vi "Configure Channel Output.vi"(0 "VISA resource name":refnum<visa-resource-name>, 1 "Output Impedance (50 Ohm)":dbl=50.0, 2 "High Voltage Limit (5 V)":dbl=5.0, 3 "Output Polarity (0: Normal)":i32(ring) items=["Normal", "Inverted"], 5 "Channel (1: 1)":i32(ring)=1 items=["1"=1, "2"=2], 9 "Output State (0: Normal)":i32(ring) items=["Normal", "Gated"], 11 "error in (no error)":errorcluster, 12 "Enable Output (T: Enable)":bool=TRUE, 13 "Low Voltage Limit (-5 V)":dbl=-5.0, 14 "Enable Voltage Limit (T: Enable)":bool=TRUE) -> (4 "VISA resource name out":refnum<visa-resource-name>, 15 "error out":errorcluster)   [LabVIEW 2018, in "AWG.lvlib" / "Agilent 3352X Series.lvlib"]
doc: "Configure output impedance, polarity, state and voltage limitation for specified channel."
uses:
  Agilent 3352X Series.lvlib
panel:
  # "Voltage Limit"
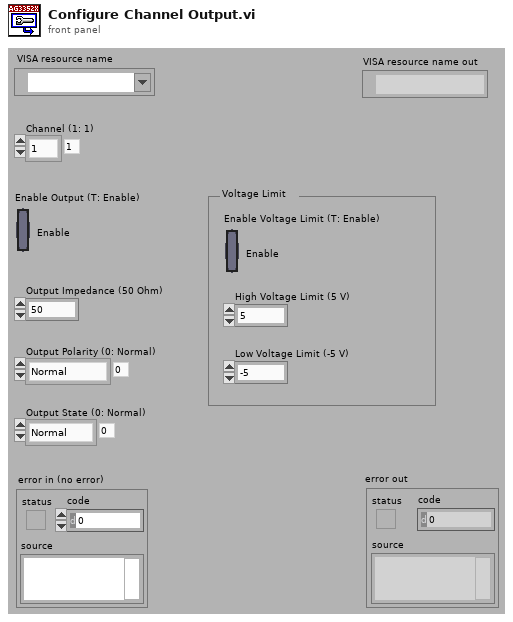
[diagram p1: front panel]
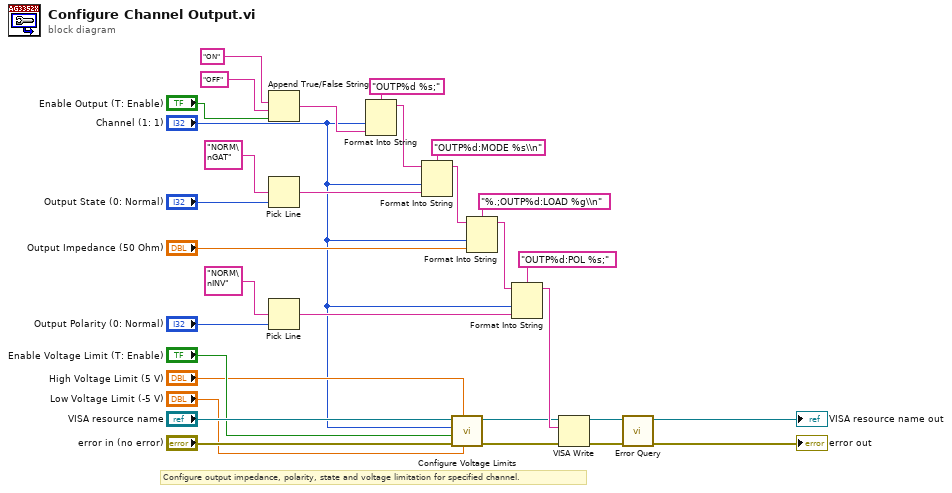
[diagram p0: block diagram]
diagram:
  # "Configure output impedance, polarity, state and voltage limitation for specified channel."
  n1 = Append True/False String(1:"Enable Output (T: Enable)", 2:"OFF", 3:"ON") -> (0:w8:string)  [unwired: 1 out]
  n2 = Pick Line(multi-line string="NORM\nGAT", line index="Output State (0: Normal)") -> (output string=w12:string)  [unwired: 1 out]
  n3 = Pick Line(multi-line string="NORM\nINV", line index="Output Polarity (0: Normal)") -> (output string=w25:string)  [unwired: 1 out]
  n4 = Format Into String(format string="OUTP%d %s;", "Channel (1: 1)", w8) -> (resulting string=w3:string)  [unwired: 2 in, 1 out]
  n5 = Format Into String(format string="OUTP%d:MODE %s\\n", initial string=w3, "Channel (1: 1)", w12) -> (resulting string=w26:string)  [unwired: 1 in, 1 out]
  n6 = call "Configure Voltage Limits.vi"("Low Voltage Limit (-5 V)"="Low Voltage Limit (-5 V)", "High Voltage Limit (5 V)"="High Voltage Limit (5 V)", "error in (no error)"="error in (no error)", "Enable Voltage Limit (T: Enable)"="Enable Voltage Limit (T: Enable)", "Channel (1: 1)"="Channel (1: 1)", "VISA resource name"="VISA resource name") -> ("error out"=w1:errorcluster, "VISA resource name out"=w15:refnum<visa-resource-name>)  [unwired: 4 out]
  n7 = Format Into String(format string="%.;OUTP%d:LOAD %g\\n", initial string=w26, "Channel (1: 1)", "Output Impedance (50 Ohm)") -> (resulting string=w22:string)  [unwired: 1 in, 1 out]
  n8 = Format Into String(format string="OUTP%d:POL %s;", initial string=w22, "Channel (1: 1)", w25) -> (resulting string=w21:string)  [unwired: 1 in, 1 out]
  n9 = VISA Write(VISA resource name=w15, write buffer=w21, error in (no error)=w1) -> (VISA resource name out=w17:refnum<visa-resource-name>, error out=w19:errorcluster)  [unwired: 1 out]
  n10 = call "Error Query.vi"("error in (no error)"=w19, "VISA resource name"=w17) -> ("error out"=→"error out":errorcluster, "VISA resource name out"=→"VISA resource name out":refnum<visa-resource-name>)  [unwired: 8 out]
